vi "Make unpersistent.vi"(8 "error in (no error)":errorcluster, 11 "PS Driver with Persistence in":refnum<class "PS Driver with Persistence.lvclass">) -> (0 "error out":errorcluster, 3 "PS Driver with Persistence out":refnum<class "PS Driver with Persistence.lvclass">)   [LabVIEW 2020, in "PS Driver.lvlib" / "PS Driver with Persistence.lvclass"]
uses:
  PS Driver with Persistence.lvclass
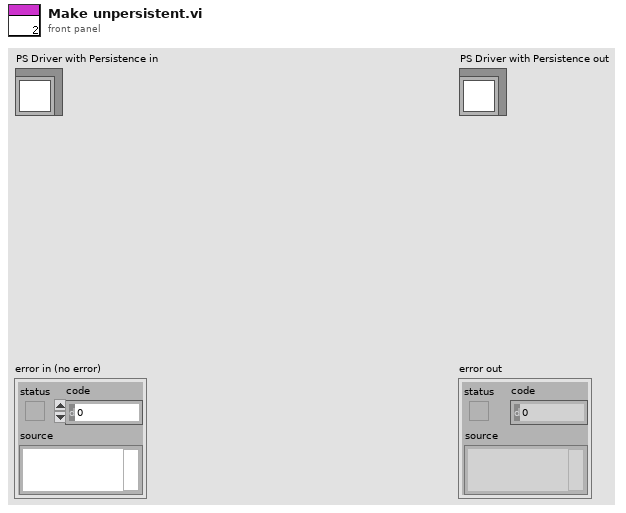
[diagram p1: front panel]
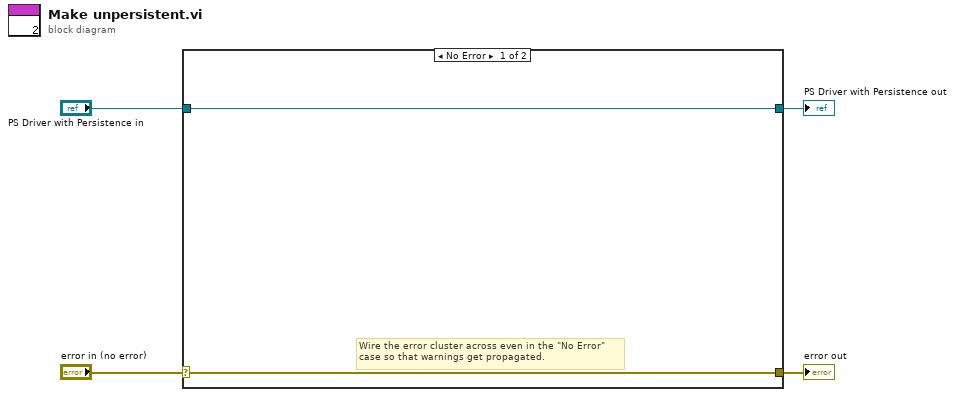
[diagram p0: block diagram]
diagram:
  n1 = case shown="No Error" "error in (no error)" {
    selector: "error in (no error)" -> [w5 w8]
    tunnel: [w5 w8] -> w3
    tunnel: [w6 w7] -> w1
    tunnel: "PS Driver with Persistence in" -> [w6 w7]
    frame No Error {
      # "Wire the error cluster across even in the \"No Error\"\ncase so that warnings get propagated."
    }
    frame Error {
    }
  }
  "error out" <- w3
  "PS Driver with Persistence out" <- w1
